vi "uMsg Get ACK.vi"(8 "error in (no error)":errorcluster, 11 "uMsg in":refnum<class "uMsg.lvclass">) -> (0 "error out":errorcluster, 2 "ACK":bool, 3 "uMsg out":refnum<class "uMsg.lvclass">)   [LabVIEW 2023, in "uLib.lvlib" / "uMsg.lvclass"]
doc: "Read the 'ACK' tag when receiving a reply message to identify whether or not the original message has been processed successfully."
uses:
  uMsg.lvclass
  uMsg.lvclass/uMsg.ctl
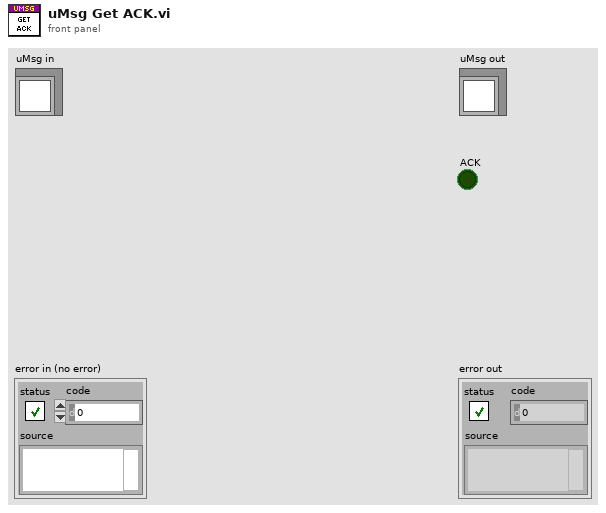
[diagram p1: front panel]
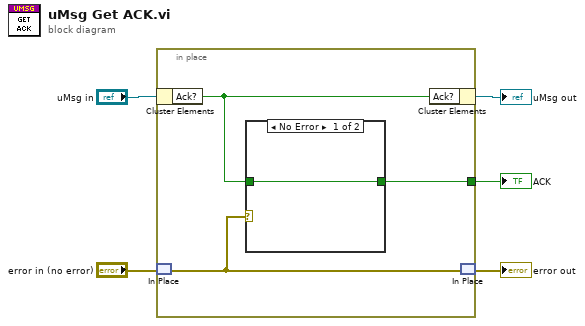
[diagram p0: block diagram]
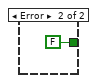
[diagram p2: hidden frame]
diagram:
  n1 = in-place {
    in-place-border: [w8] -> w5
    n2 = in-place-cluster #1("uMsg in") -> ("Ack?"=w7:bool)
    n3 = in-place-match #2("error in (no error)") -> (w6:errorcluster)
    n4 = case shown="No Error" w6 {
      tunnel: w7 -> [w9 _]
      tunnel: [w9 FALSE ("Ack?")] -> w8
      frame No Error {
      }
      frame Error {
      }
    }
    n5 = in-place-cluster #1("Ack?"=w7) -> (→"uMsg out":refnum<class "uMsg.lvclass">)
    n6 = in-place-match #2(w6) -> (→"error out":errorcluster)
  }
  "ACK" <- w5
